vi "Configure Auxiliary Input.vi"(0 "VISA resource name":refnum<visa-resource-name>, 1 "Auxiliary Input Auto Range (F: Disable)":bool, 2 "Scaling Factor (1.0000)":dbl=1.0 min=0.0001 max=99999.9999 format="%.4f", 3 "Auxiliary Input Number (1)":i32(ring)=1 items=["1"=1, "2"=2], 5 "Auxiliary Input Manual Range (20V)":dbl(ring)=20.0 items=["50m"=0.05, "100m"=0.1, "200m"=0.2, "500m"=0.5, "1"=1.0, "2"=2.0, "5"=5.0, "10"=10.0, "20"=20.0], 7 "Linear Scale A (1.000)":dbl=1.0 min=0.001 max=1000000.0 format="%.3g", 9 "Linear Scale B (0.000)":dbl min=-1000000.0 max=1000000.0 format="%.3g", 11 "error in (no error)":errorcluster, 12 "Auxiliary Input Line Filter (0: OFF)":i32(ring) items=["OFF", "100", "1000"]) -> (4 "VISA resource name out":refnum<visa-resource-name>, 15 "error out":errorcluster)   [LabVIEW 2021, in "Yokogawa WT1800 Series.lvlib"]
doc: "Configures the auxiliary input features.\nYou can apply the signals of sensors, such as luminance, wind-power, or temperature sensors, to the AUX1 and AUX2 connectors, and display the physical values measured by the sensors.\n\n<b>Note:</b>\nThis VI is only valid on models with the auxiliary input (/AUX) option."
uses:
  <instrlib>/Yokogawa WT1800 Series/Yokogawa WT1800 Series.lvlib
panel:
  # "V"
  # "Hz"
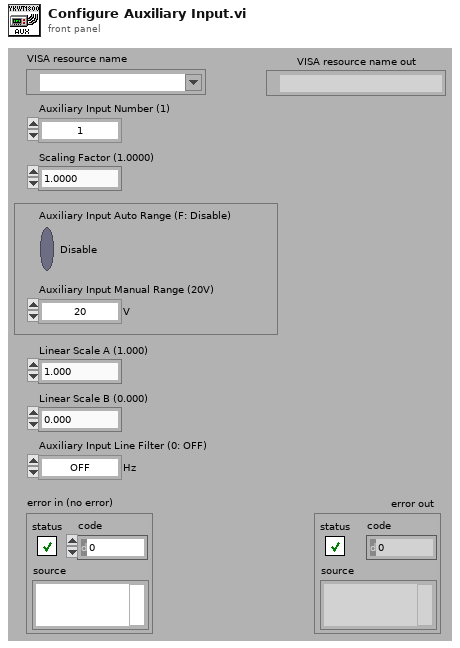
[diagram p1: front panel]
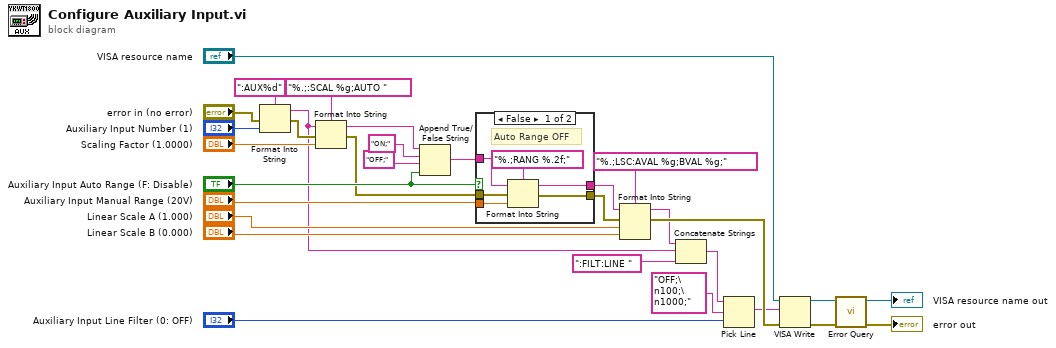
[diagram p0: block diagram]
diagram:
  n1 = Format Into String(format string=":AUX%d" ("形式文字列"), error in="error in (no error)", "Auxiliary Input Number (1)") -> (resulting string=w2:string, error out=w5:errorcluster)  [unwired: 1 in]
  n2 = Format Into String(format string="%.;:SCAL %g;AUTO " ("形式文字列"), initial string=w2, error in=w5, "Scaling Factor (1.0000)") -> (resulting string=w3:string, error out=w6:errorcluster)
  n3 = Append True/False String ("True/False 文字列を追加")(1:"Auxiliary Input Auto Range (F: Disable)", 2:"OFF;", 3:"ON;", 4:w3) -> (0:w18:string)
  n4 = case shown="False" "Auxiliary Input Auto Range (F: Disable)" {
    tunnel: w18 -> [w36 w38]
    tunnel: "Auxiliary Input Manual Range (20V)" -> [w35 _]
    tunnel: w6 -> [w34 w39]
    tunnel: [w33 w39] -> w14
    tunnel: [w32 w38] -> w13
    frame False {
      # "Auto Range OFF"
      n5 = Format Into String(format string="%.;RANG %.2f;" ("形式文字列"), initial string=w36, error in=w34, w35) -> (resulting string=w32:string, error out=w33:errorcluster)
    }
    frame True {
      # "Auto Range ON"
    }
  }
  n6 = Format Into String(format string="%.;LSC:AVAL %g;BVAL %g;" ("形式文字列"), initial string=w13, error in=w14, "Linear Scale A (1.000)", "Linear Scale B (0.000)") -> (resulting string=w11:string, error out=w21:errorcluster)
  n7 = Concatenate Strings(w11, w2, ":FILT:LINE " ("形式文字列")) -> (w10:string)
  n8 = Pick Line ("ライン選択")(string ("")=w10, multi-line string="OFF;\n100;\n1000;" ("複数行文字列"), line index="Auxiliary Input Line Filter (0: OFF)") -> (output string=w1:string)
  n9 = VISA Write ("VISA書き込み")(VISA resource name="VISA resource name", write buffer=w1, error in (no error)=w21) -> (VISA resource name out=w31:refnum<visa-resource-name>, error out=w30:errorcluster)  [unwired: 1 out]
  n10 = call <instrlib>:"Error Query.vi"("error in (no error)"=w30, "VISA resource name"=w31) -> ("error out"=→"error out":errorcluster, "VISA resource name out"=→"VISA resource name out":refnum<visa-resource-name>)  [unwired: 6 in, 2 out]
